vi "Extract Product (subVI).vi"(9 "Product name":string, 11 "Data Cluster":T1) -> (3 "Data cluster output":T1)   [LabVIEW 2020, in "Stock.lvlib"]
uses:
  Stock.lvlib
  Module Data--cluster.ctl
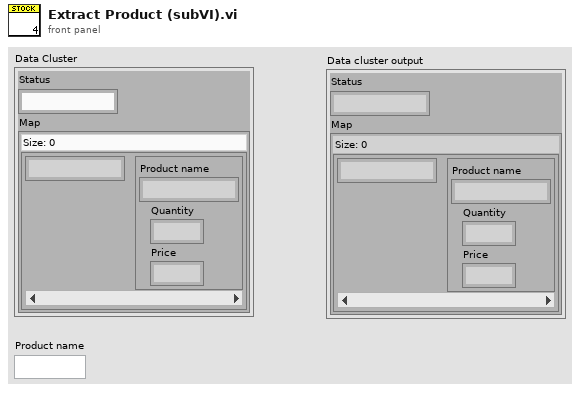
[diagram p1: front panel]
types:
  T1 = typedef "Stock.lvlib/Module Data--cluster.ctl" = cluster{"Status":string, "Map":map{string, cluster{"Product name":string, "Quantity":dbl, "Price":dbl}}}
  T2 = map{string, cluster{"Product name":string, "Quantity":dbl, "Price":dbl}}
  T3 = cluster{"Product name":string, "Quantity":dbl, "Price":dbl}
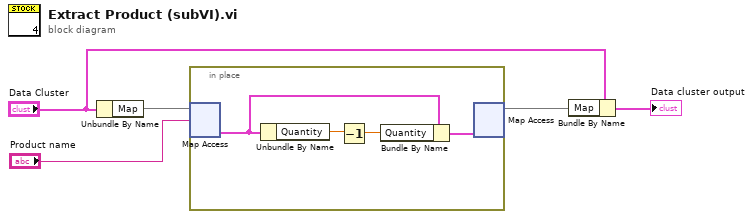
[diagram p0: block diagram]
diagram:
  n1 = Unbundle By Name("Data Cluster") -> ("Map"=w5:T2)
  n2 = in-place {
    n3 = in-place-map #1(w5, "Product name") -> (w6:T3)  [unwired: 1 in, 1 out]
    n4 = Unbundle By Name(w6) -> ("Quantity"=w9:dbl)
    n5 = Decrement(x=w9) -> (x-1=w7:dbl)
    n6 = Bundle By Name(cluster=w6, "Quantity"=w7) -> (w8:T3)
    n7 = in-place-map #1(w8) -> (w2:T2)  [unwired: 1 in, 2 out]
  }
  n8 = Bundle By Name(cluster="Data Cluster", "Map"=w2) -> (→"Data cluster output":T1)
